vi "MainStateMachine.vi"() -> ()   [LabVIEW 2018]
uses:
  Type_Def_Current_state_output.ctl
  Type_Def Actuator Controls.ctl
  <vilib>/Platform/TimedLoop/XDataNode/timing_clust.ctl
  <vilib>/Platform/TimedLoop/XDataNode/nitl_modes.ctl
  <vilib>/Platform/TimedLoop/XDataNode/wakeup.ctl
  <vilib>/Platform/TimedLoop/XDataNode/loadnilvce.vi
  <vilib>/platform/TimedLoop/XDataNode/XDataNode.xnode
  <vilib>/Platform/TimedLoop/XDataNode/XDNodeRunTimeDep.lvlib
panel:
  in  "error constant":errorcluster
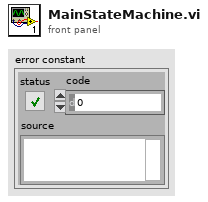
[diagram p1: front panel]
types:
  T1 = typedef "Type_Def Actuator Controls.ctl" = cluster{"Reverse ":bool, "Forward":bool, "Low Side":bool, "Precharge":bool, "High Side":bool, "Digital Out 5":bool, "Digital Out 6":bool, "Digital Out 7 ":bool, "24 Power":bool, "Tank Valve ":bool, "Brake Valve":bool, "Pump":bool, "Digital Out 1 ":bool, "Digital Out 2":bool, "Digital Out 3":bool, "Digital Out 4 ":bool}
  T2 = typedef "Type_Def_Current_state_output.ctl" = enum16{"Blank", "Systems Check", "Idle", "Ready", "Pushing", "CrawlingPrecharge", "Braking", "Fault", "Boot Up", "Unpowered", "Crawling", "Shutdown", "Service Push", "Service Wait", "Vent", "Precharge", "Cooldown"}
  T3 = typedef "XDNodeRunTimeDep.lvlib/timing_clust.ctl" = cluster{"Expected End [f-1]":u64, "Actual End [f-1]":u64, "Finished Late? [f-1]":bool, "Expected End [i-1]":u64, "Actual End [i-1]":u64, "Finished Late? [i-1]":bool, "Expected Start [i]":u64, "Actual Start [i]":u64, "Expected Start [f]":u64, "Actual Start [f]":u64, "Source Name":string, "Structure Name":string, "Period":i64, "Deadline":i64, "Offset":i64, "Start":i64, "Priority":i32, "Timeout":i32, "Mode":T4, "Wakeup Reason":T5, "Error":errorcluster, "Source Type":string, "Secondary Source Type":string, "Global End Time":u64, "Global Start Time":u64, "Frame Duration":u64, "Iteration Duration":u64, "Assigned CPU":i32, "I/O Scan Engine Mode":u32}
  T4 = typedef "XDNodeRunTimeDep.lvlib/nitl_modes.ctl" = enum32{"No Change", "Process missed periods, maintain original phase", "Discard missed periods, maintain original phase", "Process missed periods, ignore original phase", "Discard missed periods, ignore original phase"}
  T5 = typedef "XDNodeRunTimeDep.lvlib/wakeup.ctl" = enum32{"Normal", "Aborted", "Asynchronous wakeup", "Timing source error", "Timed loop error", "Timeout"}
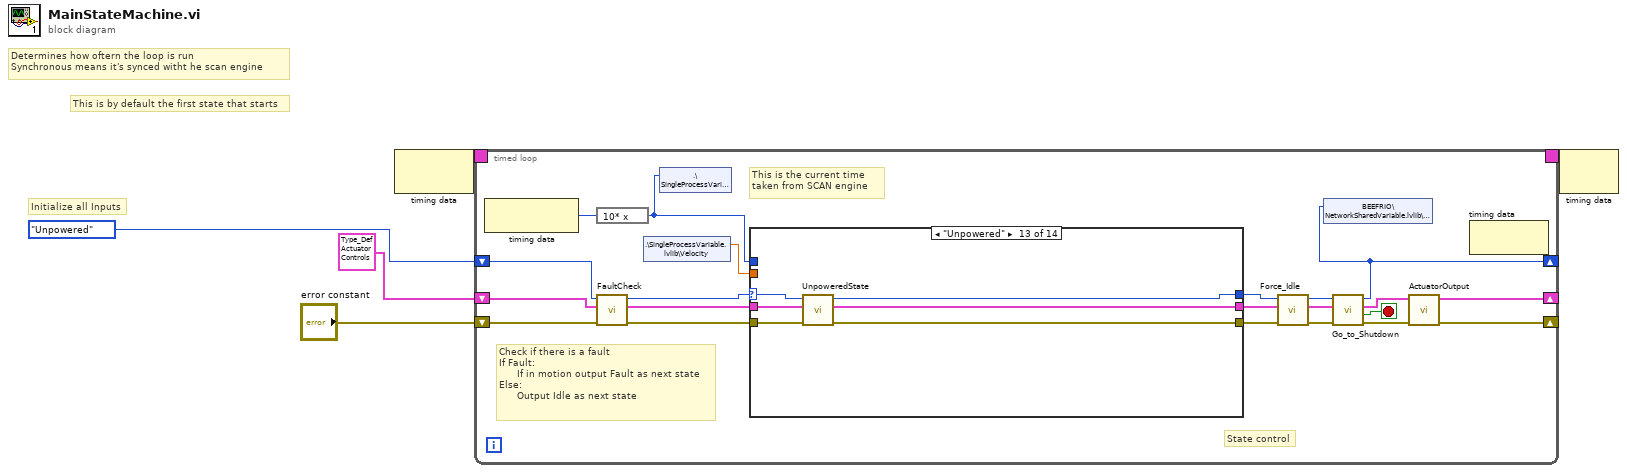
[diagram p0: block diagram]
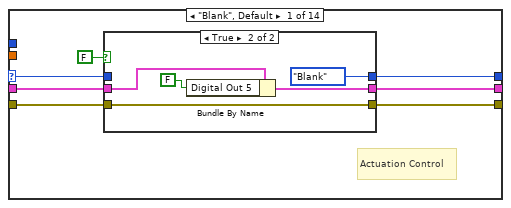
[diagram p2: hidden frame]
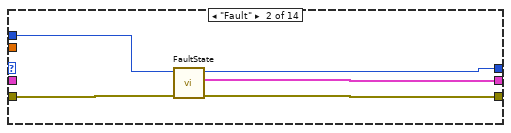
[diagram p4: hidden frame]
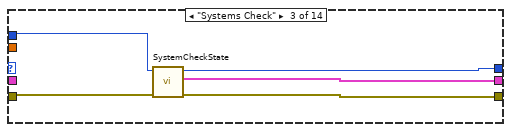
[diagram p5: hidden frame]
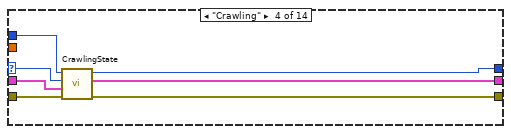
[diagram p6: hidden frame]
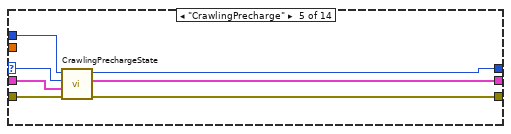
[diagram p7: hidden frame]
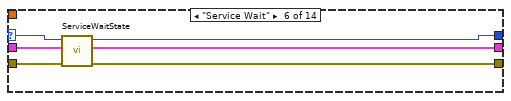
[diagram p8: hidden frame]
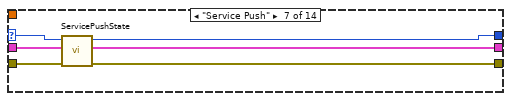
[diagram p9: hidden frame]
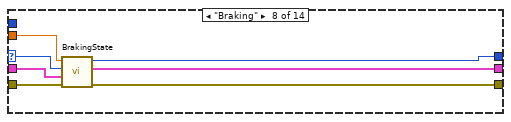
[diagram p10: hidden frame]
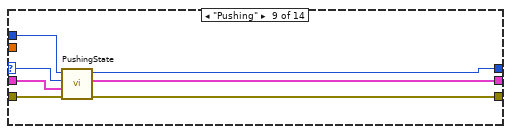
[diagram p11: hidden frame]
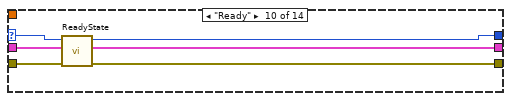
[diagram p12: hidden frame]
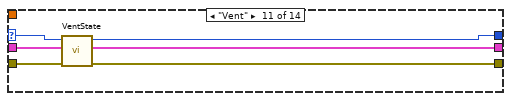
[diagram p13: hidden frame]
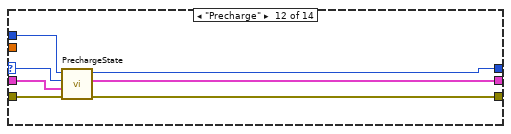
[diagram p14: hidden frame]
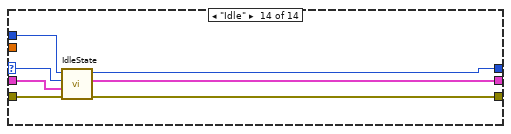
[diagram p15: hidden frame]
diagram:
  # "Determines how oftern the loop is run \nSynchronous means it's synced witht he scan engine"
  # "Initialize all Inputs"
  # "This is by default the first state that starts"
  n1 = node-c288() -> (w5:T3)  [unwired: 1 in]
  n2 = timed-loop {
    timing: w5 -> [_]
    timing-out: [_] -> w4
    shift-right: [w6] -> _
    shift-left: Type_Def_Current_state_output."Unpowered" -> [w26]
    shift-right: [w12] -> _
    shift-left: T1 {"Reverse "=FALSE, "Forward"=FALSE, "Low Side"=FALSE, "Precharge"=FALSE, "High Side"=FALSE, "Digital Out 5"=FALSE, "Digital Out 6"=FALSE, "Digital Out 7 "=FALSE, "24 Power"=FALSE, "Tank Valve "=FALSE, "Brake Valve"=FALSE, "Pump"=FALSE, "Digital Out 1 "=FALSE, "Digital Out 2"=FALSE, "Digital Out 3"=FALSE, "Digital Out 4 "=FALSE} -> [w25]
    shift-right: [w11] -> _
    shift-left: "error constant" -> [w24]
    stop <- w15 stop-if-true
    # "Check if there is a fault\nIf Fault:\n      If in motion output Fault as next state\nElse:\n      Output Idle as next state"
    # "This is the current time \ntaken from SCAN engine"
    # "State control"
    n3 = node-c288() -> (w14:i64)  [unwired: 1 in]
    n4 = expression code="10* x"(w14) -> (w13:i64)
    n5 = call "FaultCheck.vi"("error in (no error)"=w24, "Cluster in"=w25, "Enum in"=w26) -> ("error out"=w7:errorcluster, "Cluster out"=w8:T1, "Enum out"=w9:T2)  [unwired: 6 in]
    n6 = shared-variable ".\\SingleProcessVariable.lvlib\\Velocity"() -> (w10:dbl)  [unwired: 1 in, 1 out]
    n7 = shared-variable ".\\SingleProcessVariable.lvlib\\Time"(w13) -> ()  [unwired: 1 in, 1 out]
    n8 = case shown="\"Unpowered\"" w9 {
      selector: w9 -> [w33 _ _ w58 w65 w71 w77 w84 w91 w97 w103 w110 w116 w123]
      tunnel: [w32 w44 w49 w57 w64 w70 w76 w83 w90 w96 w102 w109 w115 w122] -> w19
      tunnel: [w30 w42 w47 w55 w62 w68 w74 w81 w88 w94 w100 w107 w113 w120] -> w22
      tunnel: w8 -> [w31 _ _ w56 w63 w69 w75 w82 w89 w95 w101 w108 w114 w121]
      tunnel: [w29 w43 w48 w54 w61 w67 w73 w80 w87 w93 w99 w106 w112 w119] -> w20
      tunnel: w7 -> [w28 w46 w50 w53 w60 w66 w72 w79 w86 w92 w98 w105 w111 w118]
      tunnel: w13 -> [_ w45 w51 w52 w59 _ _ _ w85 _ _ w104 _ w117]
      tunnel: w10 -> [_ _ _ _ _ _ _ w78 _ _ _ _ _ _]
      frame "Blank", Default {
        # "Actuation Control"
        n9 = case shown="True" FALSE {
          tunnel: w33 -> [w36 _]
          tunnel: [w36 Type_Def_Current_state_output."Blank"] -> w32
          tunnel: w31 -> [w35 w40]
          tunnel: [w35 w38] -> w30
          tunnel: [w34 w37] -> w29
          tunnel: w28 -> [w34 w37]
          frame False {
          }
          frame True {
            n10 = Bundle By Name(cluster=w40, "Digital Out 5"=FALSE) -> (w38:T1)
          }
        }
      }
      frame "Fault" {
        n11 = call "FaultState.vi"("error in (no error)"=w46, "Actual Start [i]"=w45) -> ("error out"=w43:errorcluster, "Cluster"=w42:T1, "Numeric"=w44:i64)  [unwired: 7 in]
      }
      frame "Systems Check" {
        n12 = call "SystemCheckState.vi"("error in (no error)"=w50, "Actual Start [i]"=w51) -> ("error out"=w48:errorcluster, "Cluster"=w47:T1, "Numeric"=w49:i64)  [unwired: 7 in]
      }
      frame "Crawling" {
        n13 = call "CrawlingState.vi"("error in (no error)"=w53, "Cluster in"=w56, "Enum in"=w58, "Actual Start [i]"=w52) -> ("error out"=w54:errorcluster, "Cluster out"=w55:T1, "Enum"=w57:T2)  [unwired: 5 in]
      }
      frame "CrawlingPrecharge" {
        n14 = call "CrawlingPrechargeState.vi"("error in (no error)"=w60, "Cluster in"=w63, "Enum in"=w65, "Actual Start [i]"=w59) -> ("error out"=w61:errorcluster, "Cluster out"=w62:T1, "Enum"=w64:T2)  [unwired: 5 in]
      }
      frame "Service Wait" {
        n15 = call "ServiceWaitState.vi"("error in (no error)"=w66, "Cluster in"=w69, "Enum in"=w71) -> ("error out"=w67:errorcluster, "Cluster out"=w68:T1, "Enum"=w70:T2)  [unwired: 6 in]
      }
      frame "Service Push" {
        n16 = call "ServicePushState.vi"("error in (no error)"=w72, "Cluster in"=w75, "Enum in"=w77) -> ("error out"=w73:errorcluster, "Cluster out"=w74:T1, "Enum out"=w76:T2)  [unwired: 6 in]
      }
      frame "Braking" {
        n17 = call "BrakingState.vi"("error in (no error)"=w79, "Cluster in"=w82, "Enum in"=w84, "Double"=w78) -> ("error out"=w80:errorcluster, "Cluster"=w81:T1, "Enum"=w83:T2)  [unwired: 5 in]
      }
      frame "Pushing" {
        n18 = call "PushingState.vi"("error in (no error)"=w86, "Cluster in"=w89, "Enum in"=w91, "Actual Start [i]"=w85) -> ("error out"=w87:errorcluster, "Cluster out"=w88:T1, "Enum"=w90:T2)  [unwired: 5 in]
      }
      frame "Ready" {
        n19 = call "ReadyState.vi"("error in (no error)"=w92, "Cluster in"=w95, "Enum in"=w97) -> ("error out"=w93:errorcluster, "Cluster out"=w94:T1, "Enum"=w96:T2)  [unwired: 6 in]
      }
      frame "Vent" {
        n20 = call "VentState.vi"("error in (no error)"=w98, "Cluster in"=w101, "Enum in"=w103) -> ("error out"=w99:errorcluster, "Cluster out"=w100:T1, "Enum out"=w102:T2)  [unwired: 6 in]
      }
      frame "Precharge" {
        n21 = call "PrechargeState.vi"("error in (no error)"=w105, "Cluster in"=w108, "Enum in"=w110, "Actual Start [i]"=w104) -> ("error out"=w106:errorcluster, "Cluster out"=w107:T1, "Enum"=w109:T2)  [unwired: 5 in]
      }
      frame "Unpowered" {
        n22 = call "UnpoweredState.vi"("error in (no error)"=w111, "Cluster in"=w114, "Enum in"=w116) -> ("error out"=w112:errorcluster, "Cluster out"=w113:T1, "Enum"=w115:T2)  [unwired: 6 in]
      }
      frame "Idle" {
        n23 = call "IdleState.vi"("error in (no error)"=w118, "Cluster in"=w121, "Enum in"=w123, "Actual Start [i]"=w117) -> ("error out"=w119:errorcluster, "Cluster out"=w120:T1, "Enum"=w122:T2)  [unwired: 5 in]
      }
    }
    n24 = call "Force_Idle.vi"("error in (no error)"=w20, "Cluster in"=w22, "Enum in"=w19) -> ("error out"=w17:errorcluster, "Cluster out"=w18:T1, "Enum out"=w16:T2)  [unwired: 6 in]
    n25 = call "Go_to_Shutdown.vi"("error in (no error)"=w17, "Cluster in"=w18, "Enum in"=w16) -> ("error out"=w21:errorcluster, "Stop State Machine"=w15:bool, "Cluster out"=w23:T1, "Enum out"=w6:T2)  [unwired: 5 in]
    n26 = shared-variable "BEEFRIO\\NetworkSharedVariable.lvlib\\currentState"(w6) -> ()  [unwired: 1 in, 1 out]
    n27 = call "ActuatorOutput.vi"("error in (no error)"=w21, "Cluster in"=w23) -> ("error out"=w11:errorcluster, "Cluster"=w12:T1)  [unwired: 8 in]
    n28 = node-c288() -> ()  [unwired: 1 in, 1 out]
  }
  n29 = node-c288(w4) -> ()  [unwired: 1 out]
